vi "pixel_dwell_time_to_iterations_per_pixel.vi"(8 "error in (no error)":errorcluster, 10 "Pixel dwell time":dbl, 11 "FPGAWrapperRK110512Fiber_Spiral in":refnum<class "FPGAWrapperRK110512Fiber_Spiral.lvclass">) -> (0 "error out":errorcluster, 1 "Iterations per pixel":i32, 2 "Pixel dwell time":dbl, 3 "FPGAWrapperRK110512Fiber_Spiral out":refnum<class "FPGAWrapperRK110512Fiber_Spiral.lvclass">)   [LabVIEW 2010, in "FPGAWrapperRK110512Fiber_Spiral.lvclass"]
uses:
  FPGAWrapperRK110512Fiber_Spiral.lvclass
  FPGAWrapperRK110512Fiber_Spiral.lvclass/FPGAWrapperRK110512Fiber_Spiral.ctl
panel:
  # "[µs]"
  # "[µs]"
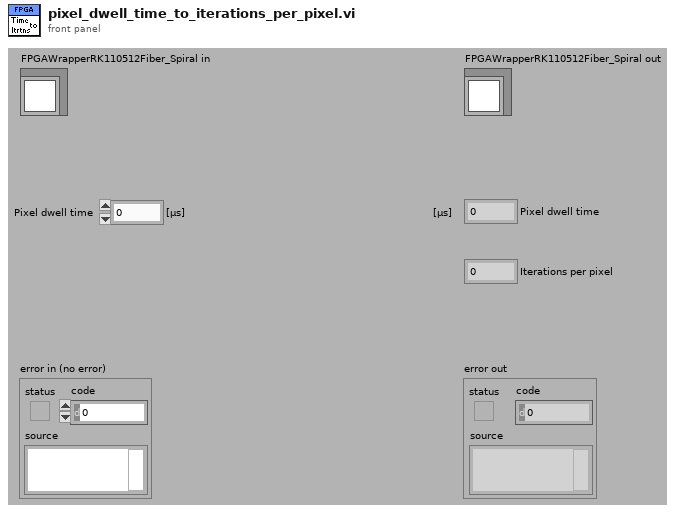
[diagram p1: front panel]
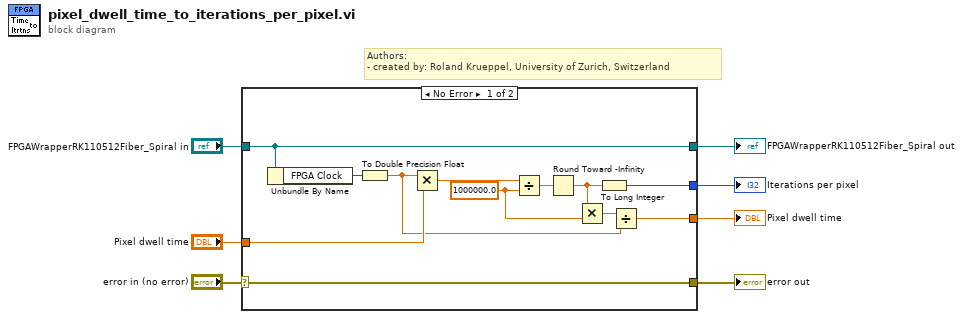
[diagram p0: block diagram]
diagram:
  # "Authors: \n- created by: Roland Krueppel, University of Zurich, Switzerland"
  n1 = case shown="No Error" "error in (no error)" {
    selector: "error in (no error)" -> [w19 w21]
    tunnel: [w19 w21] -> w6
    tunnel: [w18 w20] -> w4
    tunnel: "FPGAWrapperRK110512Fiber_Spiral in" -> [w18 w20]
    tunnel: "Pixel dwell time" -> [w17 _]
    tunnel: [w13 _] -> w2
    tunnel: [w8 _] -> w1
    frame No Error {
      w11 = 1000000.0 ("y")
      n2 = Unbundle By Name(w18) -> ("FPGA Clock"=w15:u32)
      n3 = To Double Precision Float(number=w15) -> (double precision float=w9:dbl)
      n4 = Multiply(x=w9, y=w17) -> (x*y=w16:dbl)
      n5 = Divide(x=w16, y=w11) -> (x/y=w14:dbl)
      n6 = Round Toward -Infinity(1:w14) -> (0:w12:dbl)
      n7 = Multiply(x=w12, y=w11) -> (x*y=w10:dbl)
      n8 = To Long Integer(number=w12) -> (32bit integer=w13:i32)
      n9 = Divide(x=w10, y=w9) -> (x/y=w8:dbl)
    }
    frame Error {
    }
  }
  "error out" <- w6
  "FPGAWrapperRK110512Fiber_Spiral out" <- w4
  "Pixel dwell time" <- w1
  "Iterations per pixel" <- w2
